vi "Reset Baseband Frequency Offset Phase.vi"(8 "error in (no error)":errorcluster, 11 "VISA resource name":refnum<visa-resource-name>) -> (0 "error out":errorcluster, 3 "VISA resource name out":refnum<visa-resource-name>)   [LabVIEW 2018, in "Agilent PSG MXG Series.lvlib"]
doc: "Clears the phase accumulation resulting in a phase shift of zero.\nWhen the Baseband Frequency Offset is non-zero, the hardware rotator accumulates phase-shift of the baseband signal. This residual phase remains even after the offset value is returned to zero.\nWhile there is a non-zero residual phase present in the signal, the DAC Over-Range Protection feature will automatically prevent DAC overrange errors from occurring by scaling the signal down by 1/square root of 2.\n\n<b>Note:</b>\nIt is applicable for N5172B/82B with <b>Option 004</b> only."
uses:
  Agilent PSG MXG Series.lvlib
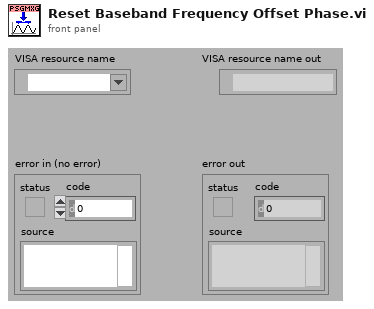
[diagram p1: front panel]
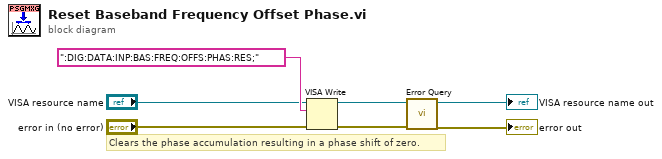
[diagram p0: block diagram]
diagram:
  # "Clears the phase accumulation resulting in a phase shift of zero."
  n1 = VISA Write(VISA resource name="VISA resource name", write buffer=":DIG:DATA:INP:BAS:FREQ:OFFS:PHAS:RES;", error in (no error)="error in (no error)") -> (VISA resource name out=w4:refnum<visa-resource-name>, error out=w3:errorcluster)  [unwired: 1 out]
  n2 = call "Error Query.vi"("error in (no error)"=w3, "VISA resource name"=w4) -> ("error out"=→"error out":errorcluster, "VISA resource name out"=→"VISA resource name out":refnum<visa-resource-name>)  [unwired: 6 in, 2 out]
